vi "CMD_DBFINDCOMP.vi"(6 "Gantry in":refnum<class "Gantry.lvclass">, 8 "error in (no error)":errorcluster, 10 "Arguments":string[](array[string]), 11 "gScript Interpreter in":refnum<class "gScript Interpreter.lvclass">) -> (0 "error out":errorcluster, 3 "gScript Interpreter out":refnum<class "gScript Interpreter.lvclass">, 4 "Gantry out":refnum<class "Gantry.lvclass">)   [LabVIEW 2023, in "gScript Interpreter.lvclass"]
uses:
  gScript Interpreter.lvclass
  Shared Components/Gantry Class/Gantry.lvclass
  Shared Components/Database/DB Component.ctl
  Shared Components/FlexWorktable/FlexWorktable.lvclass
  Shared Components/Database/Database.lvlib
panel:
  in  "Designation":u16(ring) items=["chip1", "chip2", "chip3", "chip4"]
  in  "Unstage":bool
  in  "Stage":bool
  out "Staged Components":T1(array[cluster])
  in  "finish":bool
  in  "Part Selection":string(combo)
  in  "Components":i32(listbox)
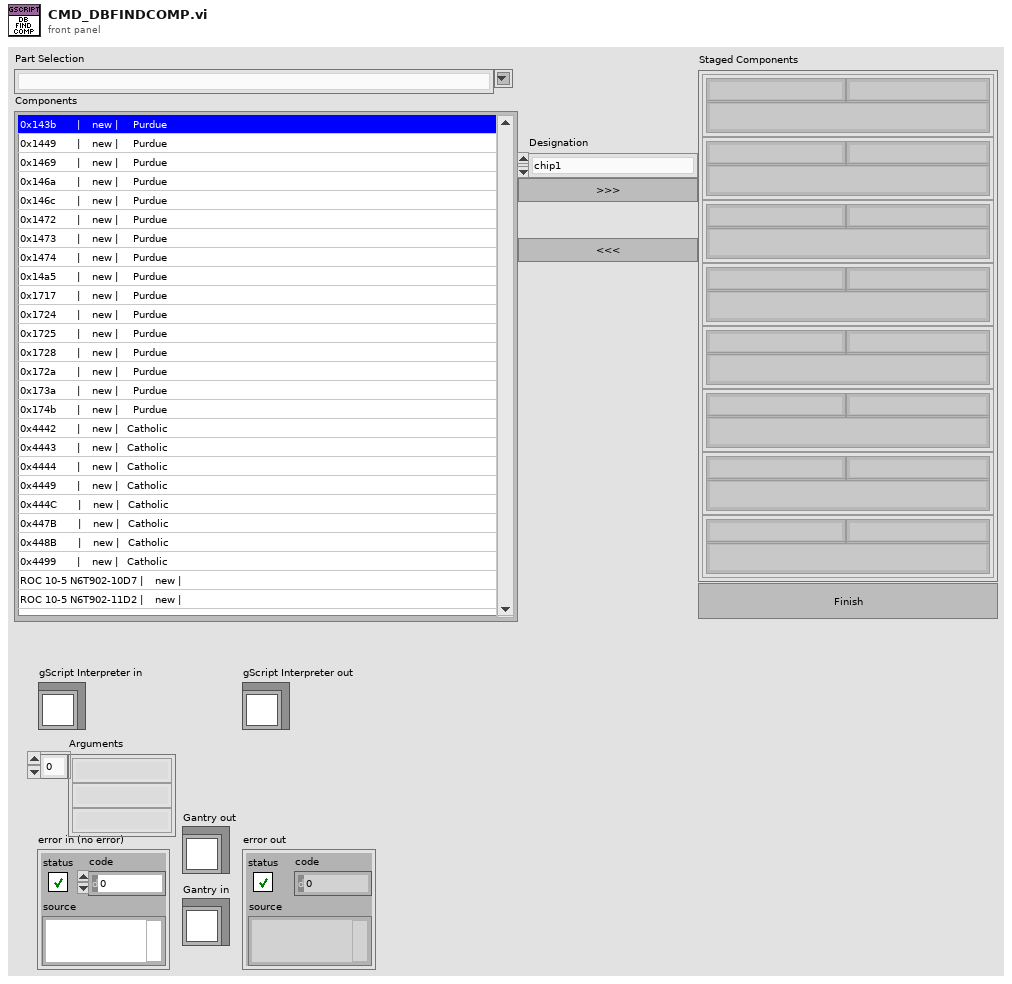
[diagram p1: front panel]
types:
  T1 = cluster{"SN":string, "Part":string, "Designation":string, "id":i32}[]
  T2 = typedef "Database.lvlib/DB Component.ctl" = cluster{"part":string, "version":i32, "id":i32, "status":string, "description":string, "serial_number":string, "location":string, "parent":i32}
  T3 = cluster{"SN":string, "Part":string, "Designation":string, "id":i32}
  T4 = typedef "Database.lvlib/DB Part.ctl" = cluster{"name":string, "description":string, "version":i32, "prefix":string, "dim_x":sgl, "dim_y":sgl, "dim_z":sgl, "type":string}
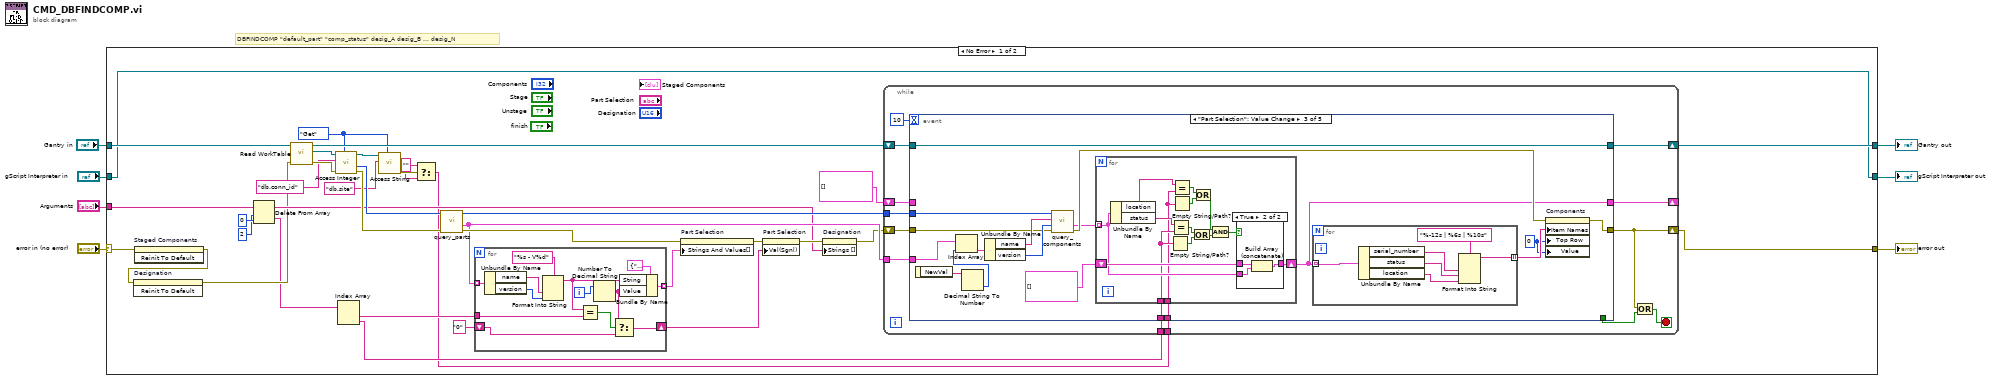
[diagram p0: block diagram]
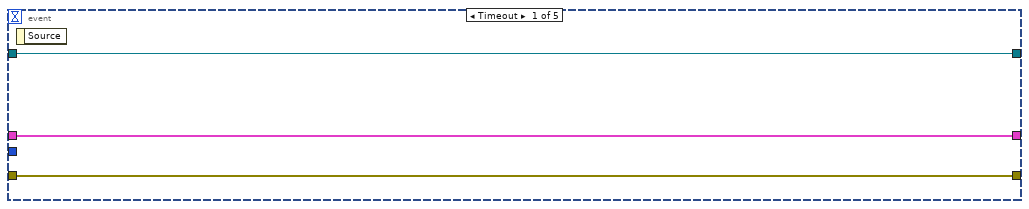
[diagram p2: hidden frame]
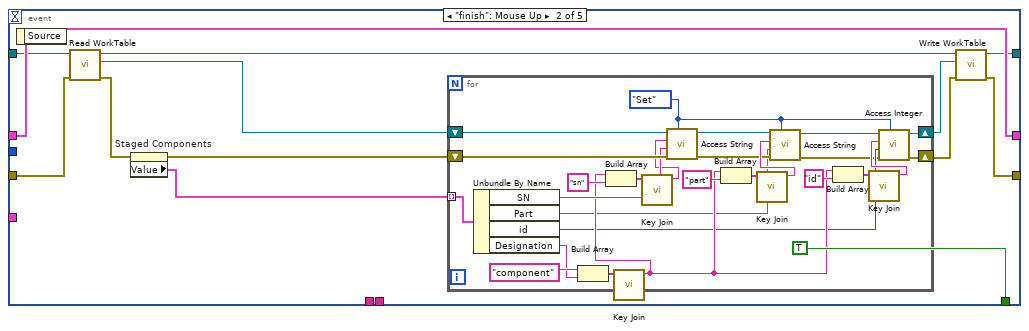
[diagram p3: hidden frame]
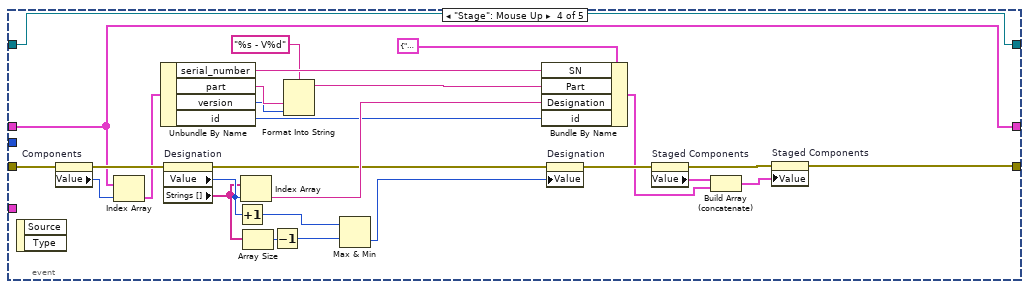
[diagram p5: hidden frame]
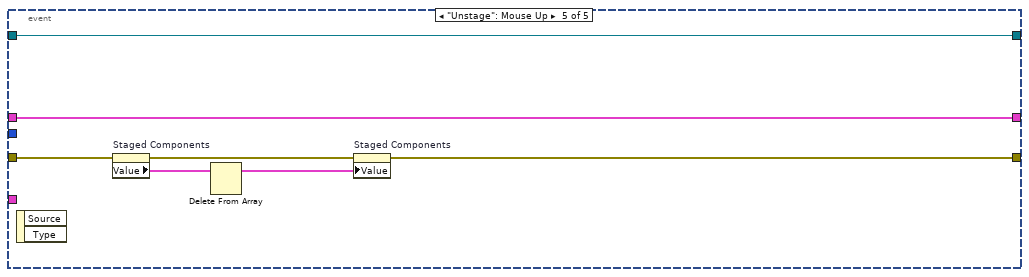
[diagram p6: hidden frame]
diagram:
  # "DBFINDCOMP \"default_part\" \"comp_status\" desig_A desig_B ... desig_N"
  n1 = case shown="No Error" "error in (no error)" {
    selector: "error in (no error)" -> [w21 w191]
    tunnel: [w30 w191] -> w6
    tunnel: [w29 w190] -> w4
    tunnel: "gScript Interpreter in" -> [w29 w190]
    tunnel: "Arguments" -> [w24 _]
    tunnel: "Gantry in" -> [w44 w189]
    tunnel: [w32 w189] -> w1
    frame No Error {
      w13 = enum16{"Get", "Set"}."Get" ("Get/Set")
      n2 = invoke on="Staged Components" class="Arr (strict)" method="Reinit To Default"(error in=w21) -> (error out=w20:errorcluster)  [unwired: 2 in, 2 out]
      n3 = invoke on="Designation" class="Ring (strict)" method="Reinit To Default"(error in=w20) -> (error out=w19:errorcluster)  [unwired: 2 in, 2 out]
      n4 = Delete From Array(array=w24, length=2, index=0) -> (deleted portion=w17:string[], array with subset deleted=w22:string[])
      n5 = call-dynamic "Read WorkTable.vi"("error in"=w19, "Gantry Class in"=w44) -> ("error out"=w42:errorcluster, "Worktable"=w43:refnum<class "FlexWorktable.lvclass">, "Gantry Class out"=w33:refnum<class "Gantry.lvclass">)  [unwired: 7 in]
      n6 = call-dynamic "Access Integer.vi"("Get/Set"=w13, "error in (no error)"=w42, "Key"="db.conn_id", "FlexWorktable in"=w43) -> ("error out"=w39:errorcluster, "Value out"=w40:i32, "FlexWorktable out"=w14:refnum<class "FlexWorktable.lvclass">)  [unwired: 5 in]
      n7 = Index Array(array=w17) -> (element #1=w16:string, element #2=w15:string)  [unwired: 2 in]
      n8 = call-dynamic "Access String.vi"("Get/Set"=w13, "Key"="db.site", "FlexWorktable in"=w14) -> ("error out"=w11:errorcluster, "Value out"=w10:string)  [unwired: 6 in, 1 out]
      n9 = Select(t="", s=w11, f=w10) -> (s? t:f=w8:string)
      n10 = call "query_parts.vi"("error in (no error)"=w39, "DB Session ID"=w40) -> ("error out"=w37:errorcluster, "Parts"=w28:T4[], "DB Session ID out"=w31:i32)  [unwired: 7 in]
      n11 = for {
        tunnel: w28 -> [w188] mode=indexing
        tunnel: [w182] -> w38 mode=indexing
        tunnel: w16 -> [w180]
        shift-right: [w177] -> w35
        shift-left: "0" -> [w178]
        i -> [w183]
        n12 = Unbundle By Name(w188) -> ("name"=w186:string, "version"=w185:i32)
        n13 = Format Into String(format string="%s - V%d", w186, w185) -> (resulting string=w181:string)  [unwired: 2 in, 1 out]
        n14 = Equal?(x=w181, y=w180) -> (x = y?=w179:bool)
        n15 = Number To Decimal String(number=w183) -> (decimal integer string=w176:string)  [unwired: 1 in]
        n16 = Select(t=w176, s=w179, f=w178) -> (s? t:f=w177:string)
        n17 = Bundle By Name(cluster=cluster{"String":string, "Value":string} {"String"="", "Value"=""}, "String"=w181, "Value"=w176) -> (w182:cluster{"String":string, "Value":string})
      }
      n18 = property on="Part Selection" class="CmbBox"(error in=w37, "Strings And Values[]"=w38) -> (error out=w34:errorcluster)  [unwired: 1 in, 1 out]
      n19 = property on="Part Selection" class="CmbBox"(error in=w34, "Val(Sgnl)"=w35) -> (error out=w26:errorcluster)  [unwired: 1 in, 1 out]
      n20 = property on="Designation" class="Ring (strict)"(error in=w26, "Strings []"=w22) -> (error out=w25:errorcluster)  [unwired: 1 in, 1 out]
      n21 = while {
        shift-right: [w56] -> w32
        shift-left: w33 -> [w57]
        shift-right: [w49] -> w30
        shift-left: w25 -> [w54]
        tunnel: w31 -> [w55]
        shift-right: [w52] -> _
        shift-left: T2[] [] ("Components") -> [w50]
        tunnel: w28 -> [w51]
        tunnel: w15 -> [w46]
        tunnel: w8 -> [w45]
        stop <- w47 stop-if-true
        n22 = event shown="[2] \"Part Selection\": Value Change" {
          selector: _ -> [_ _ _ _ _]
          dyn-events: _ -> [_ _ _ _ _]
          timeout: 10 -> [_ _ _ _ _]
          tunnel: w57 -> [w60 w71 w108 w144 w169]
          tunnel: [w60 w61 w108 w144 w169] -> w56
          tunnel: w55 -> [_ _ w117 _ _]
          tunnel: w54 -> [w59 w70 w111 w168 w175]
          tunnel: [w59 w62 w109 w158 w173] -> w49
          tunnel: [_ TRUE _ _ _] -> w48
          tunnel: [w58 w72 w101 w164 w170] -> w52
          tunnel: w51 -> [_ _ w107 _ _]
          tunnel: w50 -> [w58 w72 _ w164 w170]
          tunnel: w46 -> [_ _ w102 _ _]
          tunnel: w45 -> [_ _ w100 _ _]
          event Timeout {
            n23 = event-data() -> ()  [unwired: 1 in, 1 out]
          }
          event "finish": Mouse Up {
            n24 = event-data() -> ()  [unwired: 1 in, 1 out]
            n25 = call-dynamic "Read WorkTable.vi"("error in"=w70, "Gantry Class in"=w71) -> ("error out"=w68:errorcluster, "Worktable"=w69:refnum<class "FlexWorktable.lvclass">, "Gantry Class out"=w65:refnum<class "Gantry.lvclass">)  [unwired: 7 in]
            n26 = property on="Staged Components" class="Arr (strict)"(error in=w68) -> (error out=w67:errorcluster, "Value"=w66:T1)  [unwired: 1 in, 1 out]
            n27 = for {
              tunnel: w66 -> [w97] mode=indexing
              shift-right: [w75] -> w63
              shift-left: w67 -> [w98]
              shift-right: [w74] -> w64
              shift-left: w69 -> [w99]
              w76 = enum16{"Get", "Set"}."Set" ("Get/Set")
              n28 = Unbundle By Name(w97) -> ("SN"=w93:string, "Part"=w79:string, "id"=w78:i32, "Designation"=w92:string)
              n29 = Build Array("component" ("element"), w92) -> (w96:string[])
              n30 = call "Key Join.vi"("Key Elements"=w96) -> ("Key"=w81:string)  [unwired: 10 in]
              n31 = Build Array(w81, "sn" ("element")) -> (w94:string[])
              n32 = call "Key Join.vi"("Key Elements"=w94) -> ("Key"=w83:string)  [unwired: 10 in]
              n33 = call-dynamic "Access String.vi"("Get/Set"=w76, "error in (no error)"=w98, "Value in"=w93, "Key"=w83, "FlexWorktable in"=w99) -> ("error out"=w84:errorcluster, "FlexWorktable out"=w86:refnum<class "FlexWorktable.lvclass">)  [unwired: 4 in, 1 out]
              n34 = Build Array(w81, "part" ("element")) -> (w90:string[])
              n35 = call "Key Join.vi"("Key Elements"=w90) -> ("Key"=w85:string)  [unwired: 10 in]
              n36 = call-dynamic "Access String.vi"("Get/Set"=w76, "error in (no error)"=w84, "Value in"=w79, "Key"=w85, "FlexWorktable in"=w86) -> ("error out"=w77:errorcluster, "FlexWorktable out"=w82:refnum<class "FlexWorktable.lvclass">)  [unwired: 4 in, 1 out]
              n37 = Build Array(w81, "id" ("element")) -> (w88:string[])
              n38 = call "Key Join.vi"("Key Elements"=w88) -> ("Key"=w80:string)  [unwired: 10 in]
              n39 = call-dynamic "Access Integer.vi"("Get/Set"=w76, "error in (no error)"=w77, "Value in"=w78, "Key"=w80, "FlexWorktable in"=w82) -> ("error out"=w75:errorcluster, "FlexWorktable out"=w74:refnum<class "FlexWorktable.lvclass">)  [unwired: 4 in, 1 out]
            }
            n40 = call-dynamic "Write WorkTable.vi"("error in (no error)"=w63, "FlexWorktable"=w64, "Gantry Class in"=w65) -> ("error out"=w62:errorcluster, "Gantry Class out"=w61:refnum<class "Gantry.lvclass">)  [unwired: 7 in]
          }
          event "Part Selection": Value Change {
            w106 = 0 ("Focus Row")
            n41 = event-data() -> ("NewVal"=w116:string)  [unwired: 1 in]
            n42 = Decimal String To Number(string=w116) -> (number=w115:i32)  [unwired: 2 in, 1 out]
            n43 = Index Array(array=w107, index=w115) -> (element=w114:T4)
            n44 = Unbundle By Name(w114) -> ("name"=w113:string, "version"=w112:i32)
            n45 = call "query_components.vi"("error in (no error)"=w111, "version"=w112, "part"=w113, "DB Session ID"=w117) -> ("error out"=w105:errorcluster, "Components"=w104:T2[])  [unwired: 5 in, 1 out]
            n46 = for {
              tunnel: w104 -> [w129] mode=indexing
              tunnel: w102 -> [w126]
              shift-right: [w128] -> w101
              shift-left: T2[] [] -> [w130]
              tunnel: w100 -> [w121]
              n47 = Unbundle By Name(w129) -> ("location"=w122:string, "status"=w131:string)
              n48 = Empty String/Path?(string/path=w126) -> (empty?=w125:bool)
              n49 = Equal?(x=w131, y=w126) -> (x = y?=w127:bool)
              n50 = Empty String/Path?(string/path=w121) -> (empty?=w123:bool)
              n51 = Equal?(x=w122, y=w121) -> (x = y?=w124:bool)
              n52 = Or(x=w127, y=w125) -> (x .or. y?=w120:bool)
              n53 = Or(x=w124, y=w123) -> (x .or. y?=w119:bool)
              n54 = And(x=w119, y=w120) -> (x .and. y?=w118:bool)
              n55 = case shown="True" w118 {
                tunnel: w130 -> [w132 w135]
                tunnel: w129 -> [_ w134]
                tunnel: [w132 w133] -> w128
                frame False {
                }
                frame True {
                  n56 = Build Array (concatenate)(w135, w134) -> (w133:T2[])
                }
              }
            }
            n57 = for {
              tunnel: w101 -> [w141] mode=indexing
              tunnel: [w136] -> w110 mode=indexing
              n58 = Unbundle By Name(w141) -> ("serial_number"=w139:string, "status"=w138:string, "location"=w137:string)
              n59 = Format Into String(format string="%-12s | %6s | %10s", w139, w138, w137) -> (resulting string=w136:string)  [unwired: 2 in, 1 out]
            }
            n60 = property on="Components" class="LstBox (strict)"(error in=w105, "Item Names"=w110, "Top Row"=w106, "Value"=w106) -> (error out=w109:errorcluster)  [unwired: 1 in, 1 out]
          }
          event "Stage": Mouse Up {
            n61 = event-data() -> ()  [unwired: 1 in, 2 out]
            n62 = property on="Components" class="LstBox (strict)"(error in=w168) -> (error out=w166:errorcluster, "Value"=w167:i32)  [unwired: 1 in, 1 out]
            n63 = Index Array(array=w164, index=w167) -> (element=w162:T2)
            n64 = Unbundle By Name(w162) -> ("serial_number"=w161:string, "part"=w156:string, "version"=w155:i32, "id"=w143:i32)
            n65 = property on="Designation" class="Ring (strict)"(error in=w166) -> (error out=w153:errorcluster, "Value"=w151:u16, "Strings []"=w149:string[])  [unwired: 1 in, 1 out]
            n66 = Increment(x=w151) -> (x+1=w150:u16)
            n67 = Index Array(array=w149, index=w151) -> (element=w163:string)
            n68 = Array Size(array=w149) -> (size(s)=w148:i32)
            n69 = Decrement(x=w148) -> (x-1=w147:i32)
            n70 = Format Into String(format string="%s - V%d", w156, w155) -> (resulting string=w154:string)  [unwired: 2 in, 1 out]
            n71 = Max & Min(x=w150, y=w147) -> (min(x,y)=w146:i32)  [unwired: 1 out]
            n72 = Bundle By Name(cluster=T3 {"SN"="", "Part"="", "Designation"="", "id"=0} ("Selected Component"), "SN"=w161, "Part"=w154, "Designation"=w163, "id"=w143) -> (w142:T3)
            n73 = property on="Designation" class="Ring (strict)"(error in=w153, "Value"=w146) -> (error out=w152:errorcluster)  [unwired: 1 in, 1 out]
            n74 = property on="Staged Components" class="Arr (strict)"(error in=w152) -> (error out=w159:errorcluster, "Value"=w165:T1)  [unwired: 1 in, 1 out]
            n75 = Build Array (concatenate)(w165, w142) -> (w160:T1)
            n76 = property on="Staged Components" class="Arr (strict)"(error in=w159, "Value"=w160) -> (error out=w158:errorcluster)  [unwired: 1 in, 1 out]
          }
          event "Unstage": Mouse Up {
            n77 = event-data() -> ()  [unwired: 1 in, 2 out]
            n78 = property on="Staged Components" class="Arr (strict)"(error in=w175) -> (error out=w174:errorcluster, "Value"=w172:T1)  [unwired: 1 in, 1 out]
            n79 = Delete From Array(array=w172) -> (array with subset deleted=w171:T1)  [unwired: 2 in, 1 out]
            n80 = property on="Staged Components" class="Arr (strict)"(error in=w174, "Value"=w171) -> (error out=w173:errorcluster)  [unwired: 1 in, 1 out]
          }
        }
        n81 = Or(x=w49, y=w48) -> (x .or. y?=w47:bool)
      }
    }
    frame Error {
    }
  }
  "error out" <- w6
  "gScript Interpreter out" <- w4
  "Gantry out" <- w1
